vi "FileIO-Open Dialog.vi"(7 "Default Folder":path, 8 "error in":errorcluster, 10 "pattern (all files)":string="*.ini", 11 "Start path":path) -> (0 "error out":errorcluster, 1 "cancelled":bool, 3 "selected path":path)   [LabVIEW 2020]
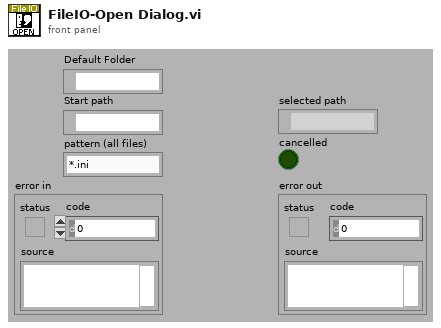
[diagram p1: front panel]
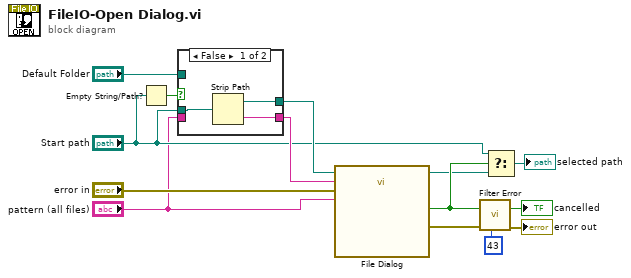
[diagram p0: block diagram]
diagram:
  n1 = Empty String/Path?(string/path="Start path") -> (empty?=w4:bool)
  n2 = case shown="False" w4 {
    tunnel: "Default Folder" -> [_ w18]
    tunnel: "Start path" -> [w16 _]
    tunnel: [w15 w18] -> w6
    tunnel: [w14 w17] -> w5
    tunnel: "pattern (all files)" -> [_ w17]
    frame False {
      n3 = Strip Path(path=w16) -> (stripped path=w15:path, name=w14:string)
    }
    frame True {
    }
  }
  n4 = call "File Dialog"("start path"=w6, "default name"=w5, "error in"="error in", "pattern (all files)"="pattern (all files)") -> ("selected path"=w8:path, "cancelled"=w9:bool, "error out"=w10:errorcluster)  [unwired: 8 in, 1 out]
  "cancelled" <- w9
  n5 = call "Filter Error.vi"("error in (no error)"=w10, "code to ignore"=43) -> ("error out"=→"error out":errorcluster)  [unwired: 9 in]
  n6 = Select(t="Start path", s=w9, f=w8) -> (s? t:f=→"selected path":path)
